vi "Constant - Maximum Analog Channel Number.vi"() -> (3 "Maximum Channel":i32=15)   [LabVIEW 2020]
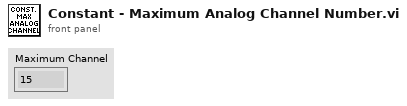
[diagram p1: front panel]
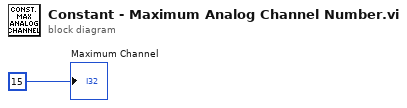
[diagram p0: block diagram]
diagram:
  "Maximum Channel" <- u16 15 ("remote port or service name")
